vi "BoundAngleNegPiToPi.vi"(1 "angle":dbl) -> (0 "bound angle":dbl)   [LabVIEW 2016]
doc: "Help by FRC Team 836 - RoboBees\nBoundAngleNegPitoPi w Help\n\nVI takes angle input and determines whether the output is 0 to Pi or -Pi to 0 degrees."
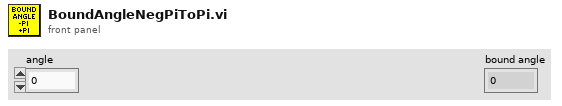
[diagram p1: front panel]
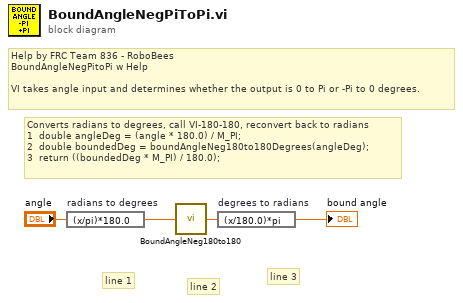
[diagram p0: block diagram]
diagram:
  # "Help by FRC Team 836 - RoboBees\nBoundAngleNegPitoPi w Help\n\nVI takes angle input and determines whether the output is 0 to Pi or -Pi to 0 degrees."
  # "line 3"
  # "line 2"
  # "line 1"
  # "Converts radians to degrees, call VI-180-180, reconvert back to radians\n1  double angleDeg = (angle * 180.0) / M_PI;\n2  double boundedDeg = boundAngleNeg180to180Degrees(angleDeg);\n3  return ((boundedDeg * M_PI) / 180.0);"
  n1 = expression code="(x/pi)*180.0" "radians to degrees"("angle") -> (w4:dbl)
  n2 = call <userlib>:"BoundAngleNeg180to180.vi"("angle"=w4) -> ("bound angle"=w3:dbl)
  n3 = expression code="(x/180.0)*pi" "degrees to radians"(w3) -> (→"bound angle":dbl)
